vi "sub vi - AI test v1.vi"(10 "stop":bool) -> (0 "error out":errorcluster, 3 "data out(DDT)":dynamicdata(waveform))   [LabVIEW 2013]
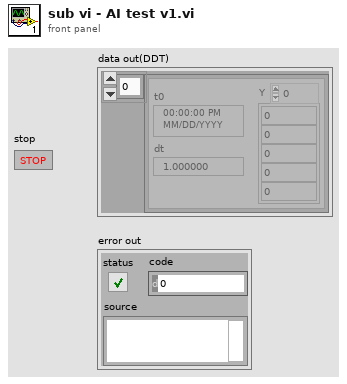
[diagram p1: front panel]
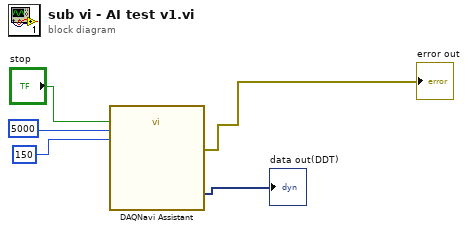
[diagram p0: block diagram]
diagram:
  n1 = call "DAQNavi Assistant"("stop(true)"="stop", "conversion rate(Hz)"=5000, "samples"=150) -> ("error out"=→"error out":errorcluster, "data out(DDT)"=→"data out(DDT)":dynamicdata)  [unwired: 23 in]
